vi "Limit Monitor.vi"(10 "Cluster":T1={"Queue Array"=[], "Queue Element"={"state"="", "data"=variant}, "System Event"=refnum, "System Event RefNum"=refnum, "Queue List"=[], "LPCA COM"="", "Rotating"=FALSE, "PrecorAI"="", "T_0 Index"=0, "Bar Graph X"=[], "Channels"=[], "Active Indicies"=[], "Active Channels"=[], "Sample Frequency"=0.0, "Ibrake Sweep"=[], "RPM Sweep"=[], "Load Sweep"=[], "Step Height Sweep"=[], "Range Sweep"=[], "A Counter"=0, "B Counter"=0, "C Counter"=0, "#A"=0, "#B"=0, "#C"=0, "Current RPM"=0.0, "Current Ibrake"=0, "Current Range"=0, "Current Step Height"=0, "Load Bank"=enum."OFF", "Cfg Cntrls"=[], "T_Monitor Indices"=[], "Thermal Limit"=0, "Thermal Resume"=0, "Timer Reset"=FALSE, "Stop Time"=0.0, "Autotest"=FALSE, "Pulsed RPM Capture"=FALSE, "Get Sample"=FALSE, "Last State"="", "Reset Timeout"=FALSE, "Ctrl Refs"={"Test Details"=refnum, "Save Config"=refnum, "Load Config"=refnum, "Path"=refnum, "Snapshot"=refnum, "SS#"=refnum, "Ibrake"=refnum, "RPM Target"=refnum, "Spin"=refnum, "Load Bank"=refnum, "Start Test"=refnum, "Pause Test"=refnum, "Load Sweep"=refnum, "RPM Sweep"=refnum, "Ibrake Sweep"=refnum, "Filters"=refnum, "Sample Frequency"=refnum, "Data Setup"=refnum, "Pause"=refnum, "Stop Time"=refnum, "S Period"=refnum, "Range"=refnum, "Step Height"=refnum, "Step Height Sweep"=refnum, "Range Sweep"=refnum, "Available Tests"=refnum, "RPM Graph"=refnum, "RPM Knob"=refnum, "FanMode"=refnum, "Fan Mode LED Array"=refnum, "Thermal Equilibrium"=refnum, "Data Display"=refnum, "LPCA Error"=refnum, "LPCA Ramp"=refnum, "LPCA Range"=refnum, "LPCA Resistance"=refnum, "Analyze Read"=refnum, "Console Select"=refnum, "Sub Panel"=refnum}, "Pulse Waveform"={"t0"=timestamp(0 s since 1904-01-01), "dt"=1.0, "Y"=[]}, "Snapshot"={"Test Details"="test", "Version"="test", "Date"=timestamp(3493915594.3018084 s since 1904-01-01), "Selected Test"="man", "Snapshot Number"=0, "Time"=timestamp(3493915602.7292905 s since 1904-01-01), "Ibrake Setpoint"="1", "RPM Setpoint"="20", "Range Setpoint"="", "Step Height Setpoint"="", "Load Bank Setpoint"="15", "Measurement Headers"="a,b,c,1,2,3", "Measurements"="1,2,3,4,5,6,7,8", "A"=0, "B"=0, "C"=0, "Raw Data"=[], "Available Tests"=enum."Manual", "Ibrake List"="", "RPM List"="", "Load Bank List"="", "Range List"="", "Step Height List"="", "FanMode Setpoint"=enum."Auto"}, "Sample Period"=0.0, "OverTemp"=FALSE, "Available Tests"=enum."Manual", "FanMode"=enum."Auto", "Fan Mode LED Array"=[FALSE, TRUE, FALSE], "Thermal\nEquilibrium "=FALSE, "Equilibrium Stop"=FALSE, "AvgDegChg"=[]} {"Snapshot"."Time" format="%<%H:%M:%S>T"; "Snapshot"."Date" format="%<%m/%d/%Y>T"}, 11 "Temperature Avg":dbl[](array[numeric])) -> (1 "Test Timer":bool caption="Time has Elapsed", 3 "Over Temp":bool, 5 "Equilibrium Stop":bool, 7 "AvgDegChg":dbl[](array[numeric]))   [LabVIEW 2017]
uses:
  Controls/Test TypeDef.ctl
  Code Library/Queue References Array.ctl
  Code Library/Queue Element.ctl
  Controls/Load Bank.ctl
  Controls/Available Tests.ctl
  Console Sim/Controls/Console Select.ctl
  Controls/Snapshot Typedef.ctl
  Controls/FanMode.ctl
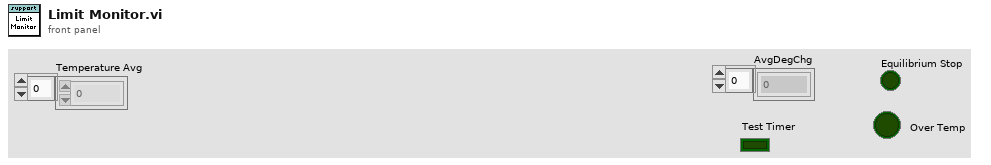
[diagram p1: front panel]
types:
  T1 = typedef "Test TypeDef.ctl" = cluster{"Queue Array":T2, "Queue Element":T3, "System Event":refnum<user-event>, "System Event RefNum":refnum<event-registration>, "Queue List":string[], "LPCA COM":refnum<visa-resource-name>, "Rotating":bool, "PrecorAI":refnum<k21>, "T_0 Index":i32, "Bar Graph X":i32[], "Channels":string[], "Active Indicies":i32[], "Active Channels":string[][], "Sample Frequency":dbl, "Ibrake Sweep":string[], "RPM Sweep":string[], "Load Sweep":string[], "Step Height Sweep":string[], "Range Sweep":string[], "A Counter":i32, "B Counter":i32, "C Counter":i32, "#A":i32, "#B":i32, "#C":i32, "Current RPM":dbl, "Current Ibrake":u32, "Current Range":u32, "Current Step Height":u32, "Load Bank":T4, "Cfg Cntrls":refnum<vi>[], "T_Monitor Indices":i32[], "Thermal Limit":i32, "Thermal Resume":i32, "Timer Reset":bool, "Stop Time":dbl, "Autotest":bool, "Pulsed RPM Capture":bool, "Get Sample":bool, "Last State":string, "Reset Timeout":bool, "Ctrl Refs":cluster{"Test Details":refnum<vi>, "Save Config":refnum<vi>, "Load Config":refnum<vi>, "Path":refnum<vi>, "Snapshot":refnum<vi>, "SS#":refnum<vi>, "Ibrake":refnum<vi>, "RPM Target":refnum<vi>, "Spin":refnum<vi>, "Load Bank":refnum<vi>, "Start Test":refnum<vi>, "Pause Test":refnum<vi>, "Load Sweep":refnum<vi>, "RPM Sweep":refnum<vi>, "Ibrake Sweep":refnum<vi>, "Filters":refnum<vi>, "Sample Frequency":refnum<vi>, "Data Setup":refnum<vi>, "Pause":refnum<vi>, "Stop Time":refnum<vi>, "S Period":refnum<vi>, "Range":refnum<vi>, "Step Height":refnum<vi>, "Step Height Sweep":refnum<vi>, "Range Sweep":refnum<vi>, "Available Tests":refnum<vi>, "RPM Graph":refnum<vi>, "RPM Knob":refnum<vi>, "FanMode":refnum<vi>, "Fan Mode LED Array":refnum<vi>, "Thermal Equilibrium":refnum<vi>, "Data Display":refnum<vi>, "LPCA Error":refnum<vi>, "LPCA Ramp":refnum<vi>, "LPCA Range":refnum<vi>, "LPCA Resistance":refnum<vi>, "Analyze Read":refnum<vi>, "Console Select":refnum<vi>, "Sub Panel":refnum<vi>}, "Pulse Waveform":waveform(dbl), "Snapshot":T5, "Sample Period":dbl, "OverTemp":bool, "Available Tests":T6, "FanMode":T7, "Fan Mode LED Array":bool[], "Thermal\nEquilibrium ":bool, "Equilibrium Stop":bool, "AvgDegChg":dbl[]}
  T2 = typedef "Queue References Array.ctl" = refnum<queue>[]
  T3 = typedef "Queue Element.ctl" = cluster{"state":string, "data":variant}
  T4 = typedef "Load Bank.ctl" = enum16{"OFF", "50", "25", "16.7", "12.5", "10.0", "8.3", "7.1", "6.3", "5.6", "5.0", "4.5", "4.2", "3.8", "3.6", "3.3", "3.1"}
  T5 = typedef "Snapshot Typedef.ctl" = cluster{"Test Details":string, "Version":string, "Date":timestamp, "Selected Test":string, "Snapshot Number":u16, "Time":timestamp, "Ibrake Setpoint":string, "RPM Setpoint":string, "Range Setpoint":string, "Step Height Setpoint":string, "Load Bank Setpoint":string, "Measurement Headers":string, "Measurements":string, "A":i32, "B":i32, "C":i32, "Raw Data":string[][], "Available Tests":T6, "Ibrake List":string, "RPM List":string, "Load Bank List":string, "Range List":string, "Step Height List":string, "FanMode Setpoint":T7}
  T6 = typedef "Available Tests.ctl" = enum16{"Manual", "EFX Brake Torque", "Generator Torque", "EFX Brake Thermal", "Generator Thermal", "Pulsed RPM", "AMT Brake Torque", "Bike Brake Torque", "AMT Brake Thermal", "Bike Brake Thermal"}
  T7 = typedef "FanMode.ctl" = enum16{"On", "Off", "Auto"}
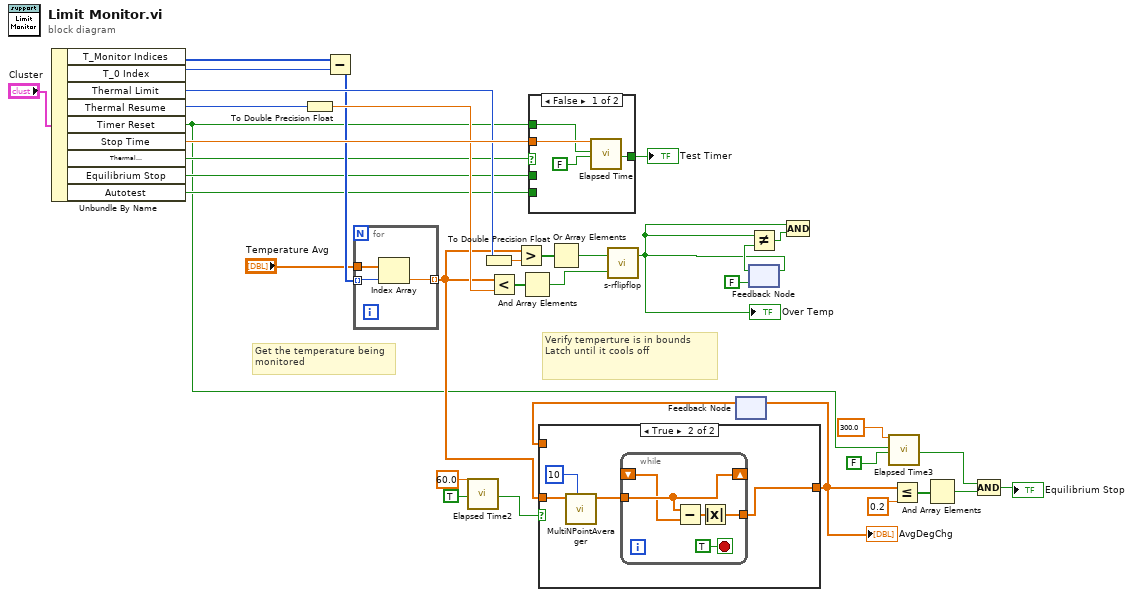
[diagram p0: block diagram]
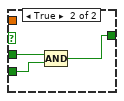
[diagram p3: hidden frame]
diagram:
  # "Get the temperature being\nmonitored"
  # "Verify temperture is in bounds\nLatch until it cools off"
  n1 = Unbundle By Name("Cluster") -> ("T_Monitor Indices"=w25:i32[], "T_0 Index"=w22:i32, "Thermal Limit"=w24:i32, "Thermal Resume"=w33:i32, "Timer Reset"=w1:bool, "Stop Time"=w35:dbl, "Thermal\nEquilibrium"=w18:bool, "Equilibrium Stop"=w17:bool, "Autotest"=w16:bool)
  n2 = To Double Precision Float(number=w33) -> (double precision float=w28:dbl)
  n3 = Subtract(x=w25, y=w22) -> (x-y=w23:i32[])
  n4 = for {
    tunnel: w23 -> [w39] mode=indexing
    tunnel: "Temperature Avg" -> [w38]
    tunnel: [w37] -> w7 mode=indexing
    n5 = Index Array(array=w38, index=w39) -> (element=w37:dbl)
  }
  n6 = call "Elapsed Time2"("Time Target (s)"=60.0, "Auto Reset"=TRUE) -> ("Time has Elapsed"=w8:bool)  [unwired: 10 in, 7 out]
  n7 = To Double Precision Float(number=w24) -> (double precision float=w34:dbl)
  n8 = Less?(x=w7, y=w28) -> (x < y?=w29:bool[])
  n9 = Greater?(x=w7, y=w34) -> (0:w32:bool[])
  n10 = And Array Elements(Boolean array=w29) -> (logical AND=w26:bool)
  n11 = case shown="False" w18 {
    tunnel: w35 -> [w42 _]
    tunnel: [w41 w44] -> w31
    tunnel: w1 -> [w40 _]
    tunnel: w17 -> [_ w45]
    tunnel: w16 -> [_ w46]
    frame False {
      n12 = call "Elapsed Time"("Time Target (s)"=w42, "Reset"=w40, "Auto Reset"=FALSE) -> ("Time has Elapsed"=w41:bool)  [unwired: 9 in, 7 out]
    }
    frame True {
      n13 = Compound Arithmetic op=AND(w45, w46) -> (w44:bool)
    }
  }
  "Test Timer" <- w31
  n14 = Or Array Elements(Boolean array=w32) -> (logical OR=w27:bool)
  n15 = call "s-rflipflop.vi"("Reset"=w26, "Set"=w27) -> ("Q"=w19:bool)  [unwired: 1 out]
  "Over Temp" <- w19
  n16 = feedback #1() -> (w6:dbl[])  [unwired: 1 in]
  n17 = case shown="True" w8 {
    tunnel: w7 -> [_ w51]
    tunnel: [w47 w48] -> w5
    tunnel: w6 -> [w47 _]
    frame False {
    }
    frame True {
      n18 = call "MultiNPointAverager.vi"("N point average"=10, "Array of values"=w51) -> ("Array of averages"=w49:dbl[])  [unwired: 9 in]
      n19 = while {
        tunnel: w49 -> [w54]
        shift-right: [w54] -> _
        shift-left: _ -> [w53]
        tunnel: [w52] -> w48
        stop <- TRUE stop-if-true
        n20 = Subtract(x=w54, y=w53) -> (x-y=w55:dbl[])
        n21 = Absolute Value(x=w55) -> (abs(x)=w52:dbl[])
      }
    }
  }
  "AvgDegChg" <- w5
  n22 = feedback-in #1(w5) -> ()
  n23 = feedback-in #2(w19) -> ()
  n24 = feedback #2(FALSE) -> (w20:bool)
  n25 = Not Equal?(x=w19, y=w20) -> (x != y?=w21:bool)
  n26 = Compound Arithmetic op=AND(w19, w21) -> ()  [unwired: 1 out]
  n27 = call "Elapsed Time3"("Time Target (s)"=300.0, "Reset"=w1, "Auto Reset"=FALSE) -> ("Time has Elapsed"=w4:bool)  [unwired: 9 in, 7 out]
  n28 = Less Or Equal?(x=w5, y=0.2) -> (x <= y?=w13:bool[])
  n29 = And Array Elements(Boolean array=w13) -> (logical AND=w12:bool)
  n30 = Compound Arithmetic op=AND(w4, w12) -> (→"Equilibrium Stop":bool)
